vi "points2contour.vi"(10 "Array":dbl[][](array[numeric]), 11 "Refnum in":T3) -> (0 "Array 2":T1(array[cluster]), 3 "Segment Information":T2(array[cluster]))   [LabVIEW 2017]
uses:
  <vilib>/vision/Image Controls.llb/IMAQ Image.ctl
  <vilib>/vision/NI_Vision_Development_Module.lvlib
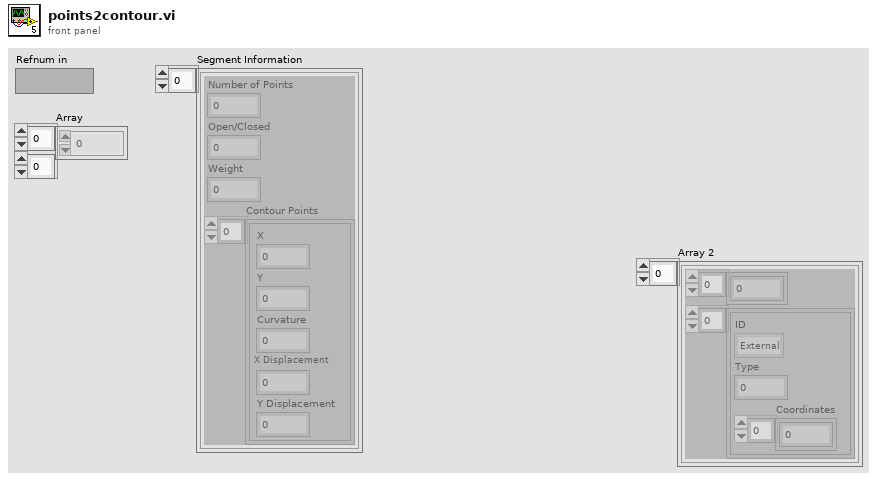
[diagram p1: front panel]
types:
  T1 = cluster{dbl[], cluster{"ID":enum32{"External", "Internal"}, "Type":u32, "Coordinates":i32[]}[]}[]
  T2 = cluster{"Number of Points":i32, "Open/Closed":i32, "Weight":dbl, "Contour Points":cluster{"X":dbl, "Y":dbl, "Curvature":dbl, "X Displacement":dbl, "Y Displacement":dbl}[]}[]
  T3 = typedef "IMAQ Image.ctl" = refnum<image>
  T4 = cluster{"ID":enum32{"External", "Internal"}, "Type":u32, "Coordinates":i32[]}
  T5 = cluster{"Area":dbl, "Number of Holes":dbl, "Bounding Rect":cluster{"Left":dbl, "Top":dbl, "Right":dbl, "Bottom":dbl}, "Center of Mass":cluster{"X":dbl, "Y":dbl}, "Orientation":dbl, "Dimensions":cluster{"Width":dbl, "Height":dbl}}[]
  T6 = cluster{"ID":enum32{"External", "Internal"}, "Type":u32, "Coordinates":i32[]}[]
  T7 = cluster{dbl[], cluster{"ID":enum32{"External", "Internal"}, "Type":u32, "Coordinates":i32[]}[]}
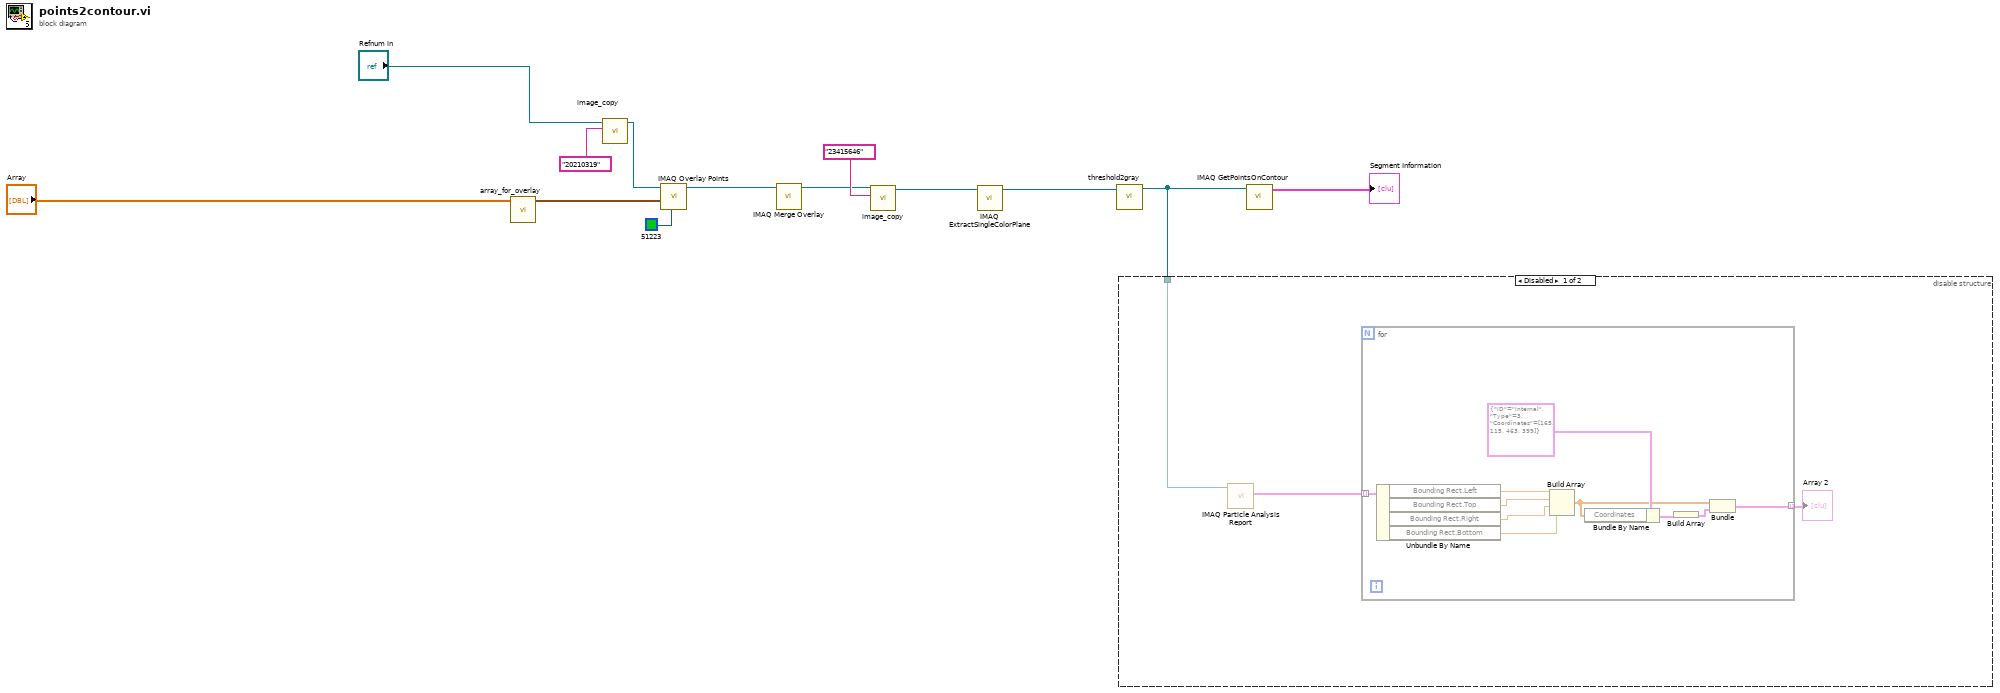
[diagram p0: block diagram]
diagram:
  n1 = call "array_for_overlay.vi"("Array in"="Array") -> ("Array out"=w11:cluster{"X":i32, "Y":i32}[])  [unwired: 10 in]
  n2 = call "image_copy.vi"("buffer name"="20210319" ("Image Name"), "image in"="Refnum in") -> ("imgae out"=w12:T3)  [unwired: 9 in]
  n3 = call "IMAQ Overlay Points"("Color"=u32 51223, "Array of Points"=w11, "Image"=w12) -> ("Image Out"=w13:T3)  [unwired: 7 in, 1 out]
  n4 = call "IMAQ Merge Overlay"("Image Src"=w13) -> ("Image Dst Out"=w6:T3)  [unwired: 9 in, 1 out]
  n5 = call "image_copy.vi"("buffer name"="23415646" ("Image Name"), "image in"=w6) -> ("imgae out"=w5:T3)  [unwired: 9 in]
  n6 = call "IMAQ ExtractSingleColorPlane"("Image Src"=w5) -> ("Image Dst Out"=w3:T3)  [unwired: 3 in, 7 out]
  n7 = call "threshold2gray.vi"("threshold image"=w3) -> ("grayscale image"=w1:T3)  [unwired: 10 in]
  n8 = disable-structure shown="Disabled" {
    disable-tunnel: w1 -> [w16 _]
    frame Disabled {
      n9 = call "IMAQ Particle Analysis Report"("Image"=w16) -> ("Particle Reports (Pixels)"=w15:T5)  [unwired: 5 in, 5 out]
      n10 = for {
        tunnel: w15 -> [w22] mode=indexing
        tunnel: [w17] -> w14 mode=indexing
        n11 = Unbundle By Name(w22) -> ("Bounding Rect.Left"=w21:dbl, "Bounding Rect.Top"=w20:dbl, "Bounding Rect.Right"=w19:dbl, "Bounding Rect.Bottom"=w18:dbl)
        n12 = Build Array(w21, w20, w19, w18) -> (w23:dbl[])
        n13 = Bundle By Name(cluster=T4 {"ID"=enum."Internal", "Type"=3, "Coordinates"=[165, 115, 463, 399]}, "Coordinates"=w23) -> (w26:T4)
        n14 = Build Array(w26) -> (w24:T6)
        n15 = Bundle(w23, w24) -> (w17:T7)  [unwired: 1 in]
      }
      "Array 2" <- w14
    }
    frame Enabled {
    }
  }
  n16 = call "IMAQ GetPointsOnContour"("Image (Edge Image)"=w1) -> ("Segment Information"=→"Segment Information":T2)  [unwired: 3 in, 2 out]
